vi "Clear Scan Time Out_3.vi"(6 "Channel number":i32, 7 "ESP32 ref":refnum<visa-resource-name>="COM4", 8 "error in (no error)":errorcluster, 11 "VISA Refnum in":refnum<visa-resource-name>) -> (0 "error out":errorcluster, 1 "error?":bool, 2 "Time out count":i32, 3 "VISA Refnum out":refnum<visa-resource-name>, 5 "ESP32 ref out":refnum<visa-resource-name>)   [LabVIEW 2023]
uses:
  <vilib>/Utility/error.llb/DialogType.ctl
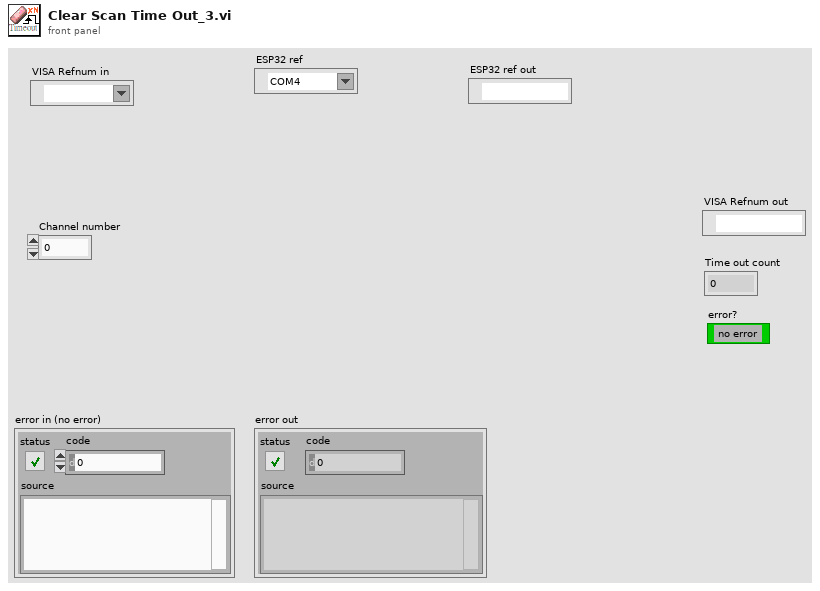
[diagram p1: front panel]
types:
  T1 = typedef "DialogType.ctl" = u16
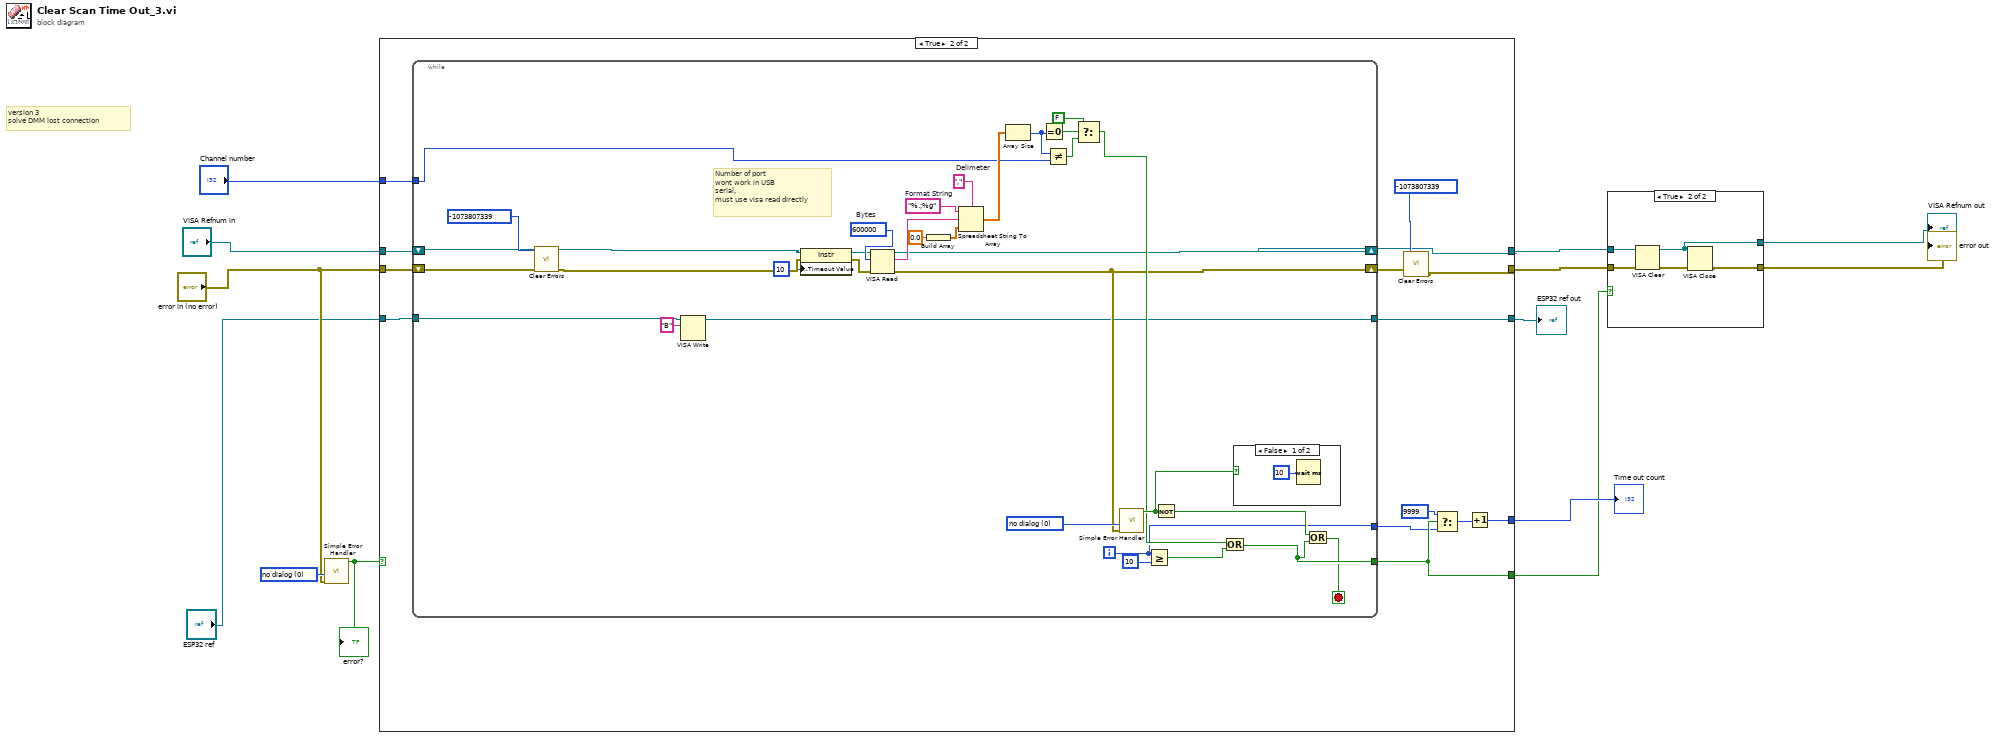
[diagram p0: block diagram]
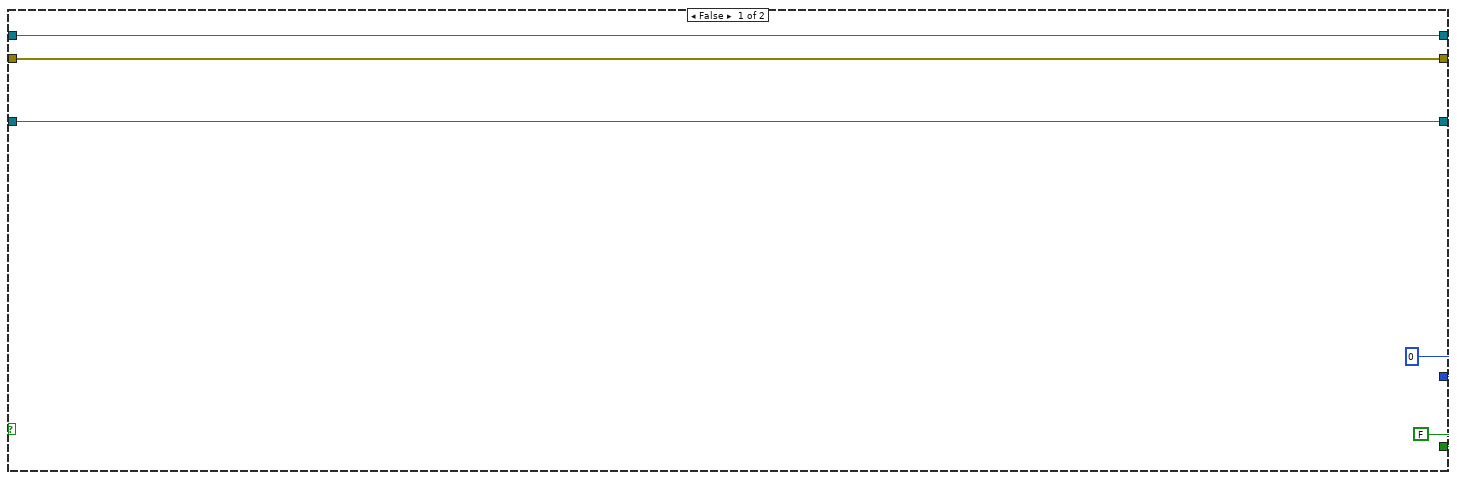
[diagram p3: hidden frame]
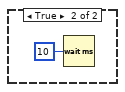
[diagram p4: hidden frame]
diagram:
  w12 = T1 0 items=["no dialog", "OK message", "continue or stop message", "OK message + warnings", "continue/stop + warnings"] ("type of dialog (OK msg:1)")
  # "version 3\nsolve DMM lost connection"
  n1 = call <vilib>:"Simple Error Handler.vi"("type of dialog (OK msg:1)"=w12, "error in (no error)"="error in (no error)") -> ("error?"=w10:bool)  [unwired: 3 in, 4 out]
  "error?" <- w10
  n2 = case shown="True" w10 {
    tunnel: [w18 w20] -> w4
    tunnel: "error in (no error)" -> [w17 w32]
    tunnel: "VISA Refnum in" -> [w18 w31]
    tunnel: [w17 w19] -> w3
    tunnel: [0 w30] -> w9
    tunnel: "ESP32 ref" -> [w16 w28]
    tunnel: [w16 w27] -> w7
    tunnel: "Channel number" -> [_ w26]
    tunnel: [FALSE w23] -> w5
    frame False {
    }
    frame True {
      n3 = while {
        shift-right: [w36] -> w25
        shift-left: w32 -> [w64]
        shift-right: [w37] -> w20
        shift-left: w31 -> [w48]
        tunnel: [w33] -> w21
        tunnel: [w43] -> w23
        tunnel: w28 -> [w47]
        tunnel: [w35] -> w27
        tunnel: w26 -> [w45]
        i -> [w33]
        stop <- w34 stop-if-true
        w56 = ","  # Delimeter
        w57 = "%.;%g"  # Format String
        w52 = u32 600000  # Bytes
        w62 = T1 0 items=["no dialog", "OK message", "continue or stop message", "OK message + warnings", "continue/stop + warnings"] ("type of dialog (OK msg:1)")
        # "Number of port\nwont work in USB \nserial,\nmust use visa read directly"
        n4 = call <vilib>:"Clear Errors.vi"("error in (no error)"=w64, "specific error code to clear (0: all)"=-1073807339 ("code out")) -> ("error out"=w63:errorcluster)  [unwired: 4 in, 1 out]
        n5 = VISA Write(VISA resource name=w47, write buffer="B") -> (VISA resource name out=w35:refnum<visa-resource-name>)  [unwired: 1 in, 2 out]
        n6 = property class="Instr"(reference=w48, error in=w63, "General Settings:Timeout Value"=u32 10) -> (reference out=w51:refnum<visa-resource-name>, error out=w50:errorcluster)
        n7 = VISA Read(VISA resource name=w51, byte count=w52, error in (no error)=w50) -> (VISA resource name out=w37:refnum<visa-resource-name>, read buffer=w53:string, error out=w36:errorcluster)  [unwired: 1 out]
        n8 = Build Array(0.0) -> (w54:dbl[])
        n9 = Spreadsheet String To Array(delimiter (Tab)=w56, format string=w57, spreadsheet string=w53, array type (2D Dbl)=w54) -> (array=w46:dbl[])
        n10 = Array Size(array=w46) -> (size(s)=w38:i32)
        n11 = Equal To 0?(x=w38) -> (x = 0?=w42:bool)
        n12 = Not Equal?(x=w38, y=w45) -> (x != y?=w41:bool)
        n13 = Select(t=FALSE, s=w42, f=w41) -> (s? t:f=w39:bool)
        n14 = call <vilib>:"Simple Error Handler.vi"("type of dialog (OK msg:1)"=w62, "error in (no error)"=w36) -> ("error?"=w59:bool)  [unwired: 3 in, 4 out]
        n15 = Greater Or Equal?(x=w33, y=10) -> (x >= y?=w44:bool)
        n16 = Not(x=w59) -> (.not. x?=w60:bool)
        n17 = Or(x=w39, y=w44) -> (x .or. y?=w43:bool)
        n18 = case shown="False" w59 {
          frame False {
            n19 = Wait (ms)(milliseconds to wait=u32 10) -> ()  [unwired: 1 out]
          }
          frame True {
            n20 = Wait (ms)(milliseconds to wait=u32 10) -> ()  [unwired: 1 out]
          }
        }
        n21 = Or(x=w60, y=w43) -> (x .or. y?=w34:bool)
      }
      n22 = call <vilib>:"Clear Errors.vi"("error in (no error)"=w25, "specific error code to clear (0: all)"=-1073807339 ("code out")) -> ("error out"=w19:errorcluster)  [unwired: 4 in, 1 out]
      n23 = Select(t=9999, s=w23, f=w21) -> (s? t:f=w29:i32)
      n24 = Increment(x=w29) -> (x+1=w30:i32)
    }
  }
  "Time out count" <- w9
  "ESP32 ref out" <- w7
  n25 = case shown="True" w5 {
    tunnel: w4 -> [w69 w73]
    tunnel: w3 -> [w68 w74]
    tunnel: [w68 w71] -> w2
    tunnel: [w69 w70] -> w1
    frame False {
    }
    frame True {
      n26 = VISA Clear(VISA resource name=w73, error in (no error)=w74) -> (VISA resource name out=w70:refnum<visa-resource-name>, error out=w72:errorcluster)
      n27 = VISA Close(VISA resource name=w70, error in (no error)=w72) -> (error out=w71:errorcluster)
    }
  }
  "error out" <- w2
  "VISA Refnum out" <- w1
